vi "am_read.vi"() -> ()   [LabVIEW 2014]
uses:
  aardvark.dll
panel:
  out "Dup Aardvark Handle":i32
  out "Data byte":u8 format="%.0x"
  out "error out":errorcluster
  in  "Memory ADD":u16=80 max=1023 format="%.0x"
  in  "Address (0x50)":u16=80 max=1023 format="%.0x"
  in  "Num Bytes to Fetch (64)":u8=64 min=1
  in  "Aardvark Handle":i32 min=0
  in  "error in (no error)":errorcluster
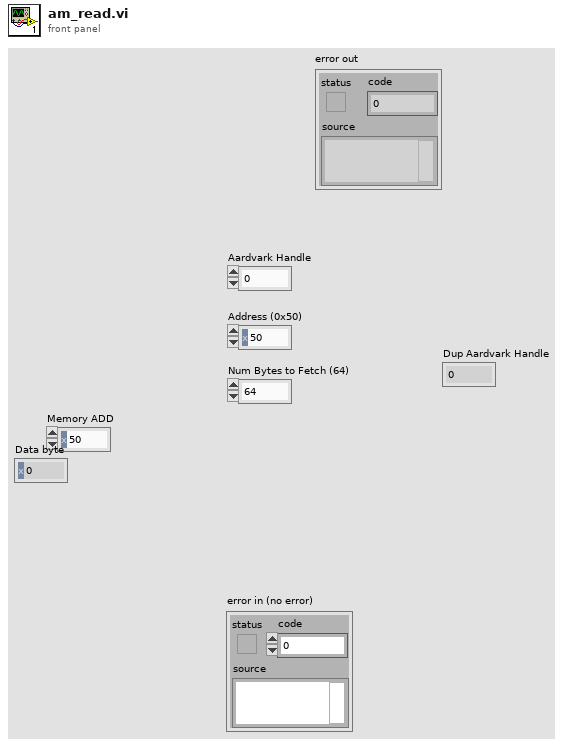
[diagram p1: front panel]
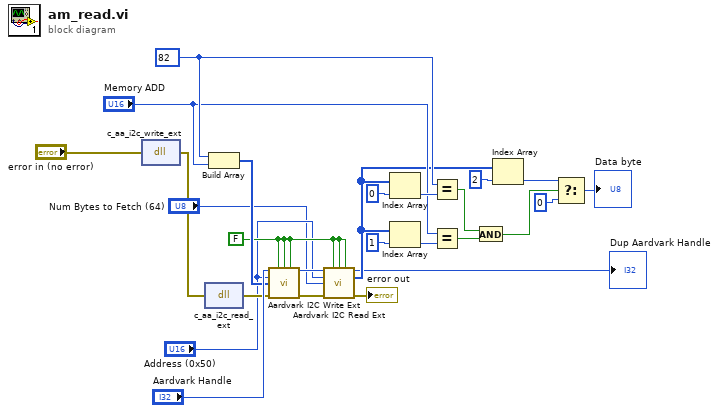
[diagram p0: block diagram]
diagram:
  w21 = FALSE
  w13 = u16 82
  n1 = dll-call lib="aardvark.dll" fn="c_aa_i2c_write_ext"(error in="error in (no error)") -> (error out=w25:errorcluster)  [unwired: 3 in, 1 out]
  n2 = dll-call lib="aardvark.dll" fn="c_aa_i2c_read_ext"(error in=w25) -> (error out=w22:errorcluster)  [unwired: 3 in, 1 out]
  n3 = Build Array(w13, "Memory ADD") -> (w23:u16[])
  n4 = call <instrlib>:"Aardvark I2C Write Ext.vi"("Aardvark Handle"="Aardvark Handle", "10-bit Addressing? (False)"=w21, "Combined Format? (False)"=w21, "No Stop? (False)"=w21, "Address (0x50)"="Address (0x50)", "Data to Write"=w23, "error in (no error)"=w22) -> ("dup Aardvark Handle"=w20:i32, "error out"=w17:errorcluster)  [unwired: 5 in, 2 out]
  n5 = call <instrlib>:"Aardvark I2C Read Ext.vi"("Aardvark Handle"=w20, "10-bit Addressing? (False)"=w21, "Combined Format? (False)"=w21, "No Stop? (False)"=w21, "Address (0x50)"="Address (0x50)", "Num Bytes to Fetch (64)"="Num Bytes to Fetch (64)", "error in (no error)"=w17) -> ("dup Aardvark Handle"=→"Dup Aardvark Handle":i32, "Incoming Data"=w2:u8[], "error out"=→"error out":errorcluster)  [unwired: 5 in, 1 out]
  n6 = Index Array(array=w2, index=0) -> (element=w14:u8)
  n7 = Index Array(array=w2, index=1) -> (element=w11:u8)
  n8 = Equal?(x=w13, y=w14) -> (x = y?=w10:bool)
  n9 = Equal?(x="Memory ADD", y=w11) -> (x = y?=w9:bool)
  n10 = And(x=w10, y=w9) -> (x .and. y?=w3:bool)
  n11 = Index Array(array=w2, index=2) -> (element=w7:u8)
  n12 = Select(t=w7, s=w3, f=u8 0) -> (s? t:f=→"Data byte":u8)
